vi "Drivetrain Loop.vi"   [LabVIEW 2014]
uses:
  Common Code/Drivetrain Status.ctl
  Drivetrain Mode.ctl
  Common Code/Dist Drive Status.ctl
  Common Code/Yaw Rate Compensation Indicators.ctl
  Common Code/Change Detect Int.vi
  Common Code/Change Detect Boolean.vi
  Robot Global Data.vi
types:
  T1 = typedef "Drivetrain Mode.ctl" = enum16{"Manual", "Gyro Steer", "Vision Steer", "Drive Distance", "Yaw Rate Compensate"}
  T2 = typedef "Drivetrain Status.ctl" = cluster{"Y (Throttle)":sgl, "X (Steer)":sgl, "Translation X":sgl, "Center Wheel Down":bool, "Mode":T1, "Distance Drive finished?":bool, "Y Target":sgl, "X Target":sgl, "Heading Target":sgl, "Dist Drive Status":T3, "Step Eject Lockout":bool, "Gyro In Range?":bool, "Yaw Comp Indicators":T4}
  T3 = typedef "Dist Drive Status.ctl" = cluster{"Y In Range":bool, "X In Range":bool, "Gyro In Range":bool, "Y Dist":dbl, "X Dist":dbl, "Gyro":dbl}
  T4 = typedef "Yaw Rate Compensation Indicators.ctl" = cluster{"Rate Command":sgl, "Rate Actual":sgl, "Steer adjustment":sgl}
  T5 = typedef "Drivetrain Control.ctl" = cluster{"Mode":T1, "Steer":dbl, "Y":dbl, "Heading Target":dbl, "Strafe X":dbl, "Y Target":dbl, "Strafe Target":dbl, "X Max Speed":dbl, "X Min Speed":dbl, "Y Max Speed":dbl, "Y Min Speed":dbl, "Force strafe":bool, "Pivot Speed":dbl}
  T6 = typedef "WPI_DriverStationRobotMode2.ctl" = enum16{"Autonomous Disabled", "Autonomous Enabled", "Teleop Disabled", "Teleop Enabled", "Disconnected", "Finish", "Test Disabled", "Test Enabled", "Emergency Stopped"}
  T7 = typedef "IMU Data.ctl" = cluster{"Pitch":sgl, "Roll":sgl, "Yaw":sgl, "Data Valid?":bool, "Temp":sgl, "MOVING":bool, "NAVX_CAL_STATUS":T8, "NAVX_OP_STATUS":T9, "YAW_STABLE":bool, "Accel X":sgl, "Accel Y":sgl, "Accel Z":sgl, "Accel Magnitude":sgl, "Pitch Rate":sgl, "Roll Rate":sgl, "Yaw Rate":sgl, "NavX Opened?":bool}
  T8 = typedef "navX-MXP IMU.lvlib/navX NAVX_CAL_STATUS.ctl" = u8
  T9 = typedef "navX-MXP IMU.lvlib/navX NAVX_OP_STATUS.ctl" = u8
  T10 = typedef "WPI_MotorControlDeviceRef.ctl" = cluster{"DeviceStatus":errorcluster, "Type":T11, "PWM":cluster{"Controller":T12, "PWM Channel":T13, "DeadBand":T14}, "CAN":cluster{"Device Number":u8, "Control Mode":T15, "Semaphore":T16, "Max Vout":dbl, "TalonSRX Control Mode":T17}, "Invert":bool, "TransformRef":T18, "InvTransformRef":T18}
  T11 = typedef "WPI_MotorControlType.ctl" = enum16{"PWM", "CAN", "CANTalonSRX"}
  T12 = typedef "FPGA_TypedefDigitalModule.ctl" = enum16{"Controller 1"}
  T13 = typedef "FPGA_DIOPWMChannel.ctl" = enum8{"PWM 0", "PWM 1", "PWM 2", "PWM 3", "PWM 4", "PWM 5", "PWM 6", "PWM 7", "PWM 8", "PWM 9", "PWM MXP 0", "PWM MXP 1", "PWM MXP 2", "PWM MXP 3", "PWM MXP 4", "PWM MXP 5", "PWM MXP 6", "PWM MXP 7", "PWM MXP 8", "PWM MXP 9", "Invalid"}
  T14 = typedef "WPI_PWMDeadband.ctl" = cluster{"Name":string, "maxPositivePwm":i32, "minPositivePwm":i32, "centerPwm":i32, "maxNegativePwm":i32, "minNegativePwm":i32, "angularRange":u16}
  T15 = typedef "WPI_CANJaguar_ControlMode.ctl" = enum8{"Percent VBus", "Current", "Speed", "Position", "Voltage"}
  T16 = typedef "Semaphore RefNum" = refnum<k1>
  T17 = typedef "WPI_CANTalonSRX_APIControlMode.ctl" = enum8{"Percent VBus", "Speed", "Position", "Slave", "Unchanged / Invalid"}
  T18 = typedef "WPI_PWMTransform_ConPane.ctl" = refnum<vi>
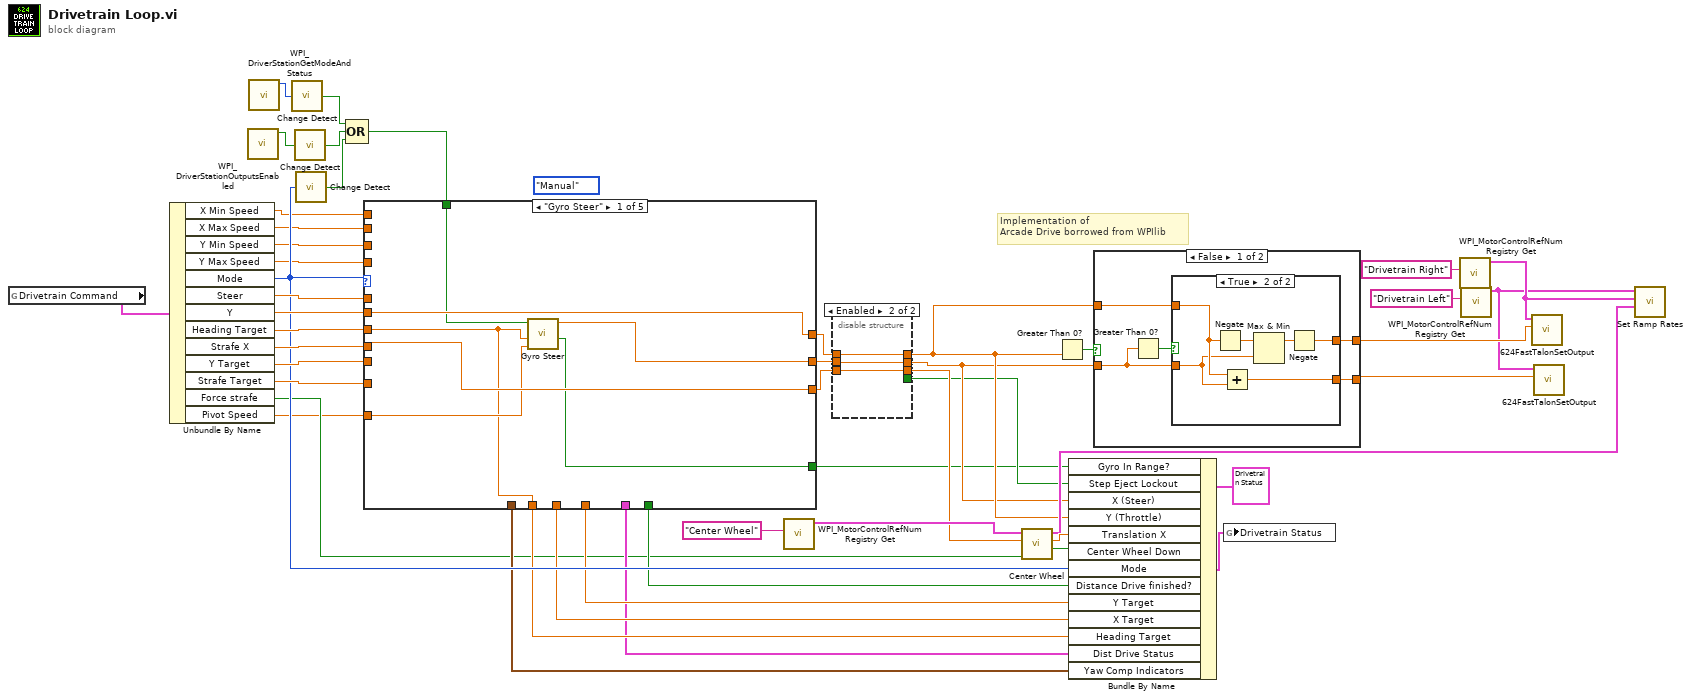
[diagram p0: block diagram]
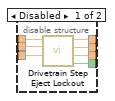
[diagram p2: hidden frame]
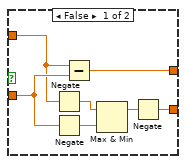
[diagram p3: hidden frame]
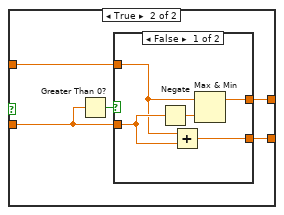
[diagram p4: hidden frame]
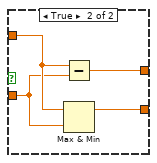
[diagram p5: hidden frame]
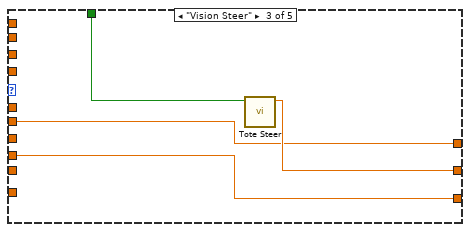
[diagram p7: hidden frame]
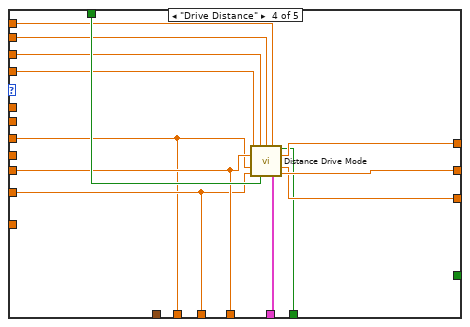
[diagram p8: hidden frame]
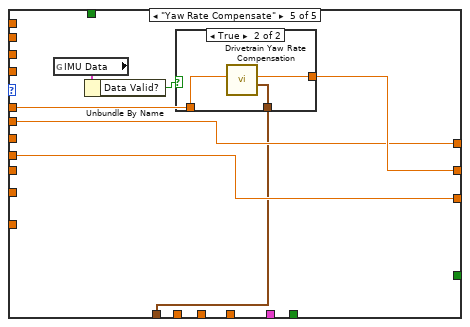
[diagram p9: hidden frame]
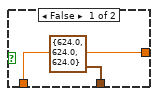
[diagram p10: hidden frame]
diagram:
  (unwired) Drivetrain_Mode."Manual" ("Mode")
  # "Implementation of \nArcade Drive borrowed from WPIlib"
  n1 = global read "Robot Global Data.vi" "Drivetrain Command"() -> (w46:T5)
  n2 = Unbundle By Name(w46) -> ("X Min Speed"=w12:dbl, "X Max Speed"=w13:dbl, "Y Min Speed"=w14:dbl, "Y Max Speed"=w15:dbl, "Mode"=w37:T1, "Steer"=w45:dbl, "Y"=w48:dbl, "Heading Target"=w47:dbl, "Strafe X"=w44:dbl, "Y Target"=w43:dbl, "Strafe Target"=w42:dbl, "Force strafe"=w2:bool, "Pivot Speed"=w1:dbl)
  n3 = call <vilib>:"WPI_DriverStationOutputsEnabled.vi"() -> ("OutputsEnabled?"=w35:bool)  [unwired: 10 in, 1 out]
  n4 = call <vilib>:"WPI_DriverStationGetModeAndStatus.vi"() -> ("Robot Mode"=w36:T6)  [unwired: 10 in, 1 out]
  n5 = call-poly "Change Detect.vi"("In"=w36) -> ("Changed?"=w32:bool)
  n6 = call-poly "Change Detect.vi"("In"=w35) -> ("Changed?"=w33:bool)
  n7 = call-poly "Change Detect.vi"("In"=w37) -> ("Changed?"=w34:bool)
  n8 = Compound Arithmetic op=OR(w32, w33, w34) -> (w31:bool)
  n9 = case shown="\"Gyro Steer\"" w37 {
    tunnel: [w54 w58 w62 w74 w81] -> w9
    tunnel: w45 -> [_ w58 _ _ w82]
    tunnel: [w55 w57 w61 w75 w80] -> w11
    tunnel: w48 -> [w55 w57 w61 _ w80]
    tunnel: w47 -> [w49 _ _ w68 _]
    tunnel: w44 -> [w53 w56 w60 _ w79]
    tunnel: [w53 w56 w60 w73 w79] -> w7
    tunnel: w43 -> [_ _ _ w70 _]
    tunnel: w42 -> [_ _ _ w69 _]
    tunnel: w31 -> [w52 _ w59 w72 _]
    tunnel: [_ _ _ w71 _] -> w30
    tunnel: [_ _ _ w70 _] -> w29
    tunnel: [_ _ _ w69 _] -> w28
    tunnel: [w49 _ _ w68 _] -> w27
    tunnel: [_ _ _ w67 _] -> w26
    tunnel: w15 -> [_ _ _ w66 _]
    tunnel: w14 -> [_ _ _ w65 _]
    tunnel: w13 -> [_ _ _ w64 _]
    tunnel: w12 -> [_ _ _ w63 _]
    tunnel: [w51 _ _ _ _] -> w4
    tunnel: [_ _ _ _ w78] -> w3
    tunnel: w1 -> [w50 _ _ _ _]
    frame "Gyro Steer" {
      n10 = call "Gyro Steer.vi"("Turn Speed"=w50, "Target Angle"=w49, "Changed?"=w52) -> ("In Range?"=w51:bool, "X out"=w54:dbl)  [unwired: 7 in]
    }
    frame "Manual", Default {
    }
    frame "Vision Steer" {
      n11 = call "Tote Steer.vi"("Changed?"=w59) -> ("f"=w62:dbl)  [unwired: 10 in]
    }
    frame "Drive Distance" {
      n12 = call "Distance Drive Mode.vi"("Y Output High"=w66, "Y Output Low"=w65, "X Output High"=w64, "X Output Low"=w63, "Y target"=w70, "Heading target"=w68, "Strafe target"=w69, "Reinitialize"=w72) -> ("isFinished"=w71:bool, "Y out"=w75:dbl, "Strafe out"=w73:dbl, "Dist Drive Status"=w67:T3, "X out"=w74:dbl)  [unwired: 3 in]
    }
    frame "Yaw Rate Compensate" {
      n13 = global read "Robot Global Data.vi" "IMU Data"() -> (w77:T7)
      n14 = Unbundle By Name(w77) -> ("Data Valid?"=w76:bool)
      n15 = case shown="True" w76 {
        tunnel: w82 -> [w84 w87]
        tunnel: [w84 w86] -> w81
        tunnel: [T4 {"Rate Command"=624.0, "Rate Actual"=624.0, "Steer adjustment"=624.0} ("Yaw Comp Indicators") w85] -> w78
        frame False {
        }
        frame True {
          n16 = call "Drivetrain Yaw Rate Compensation.vi"("Steer in"=w87) -> ("Yaw Comp Indicators"=w85:T4, "Steer Out"=w86:dbl)  [unwired: 9 in]
        }
      }
    }
  }
  n17 = call <vilib>:"WPI_MotorControlRefNum Registry Get.vi"("refnum name"="Center Wheel") -> ("MotorControlDevRef"=w19:T10)  [unwired: 9 in, 1 out]
  n18 = disable-structure shown="Enabled" {
    disable-tunnel: w11 -> [w94 w97]
    disable-tunnel: [w93 w97] -> w10
    disable-tunnel: w9 -> [w92 w96]
    disable-tunnel: [w91 w96] -> w8
    disable-tunnel: w7 -> [w90 w95]
    disable-tunnel: [w89 w95] -> w6
    disable-tunnel: [w88 _] -> w5
    frame Disabled {
      n19 = call "Drivetrain Step Eject Lockout.vi"("Strafe In"=w90, "Steer In"=w92, "Throttle In"=w94) -> ("Eject Lockout?"=w88:bool, "Strafe Out"=w89:dbl, "Steer Out"=w91:dbl, "Throttle Out"=w93:dbl)  [unwired: 5 in]
    }
    frame Enabled {
    }
  }
  n20 = call "Center Wheel.vi"("Force strafe"=w2, "Center Wheel Value"=w6, "MotorControlDevRef"=w19) -> ("Wheel Down"=w38:bool, "X Out"=w39:dbl, "MotorControlDevRef 2"=w18:T10)  [unwired: 6 in]
  n21 = Greater Than 0?(x=w10) -> (x > 0?=w25:bool)
  n22 = Bundle By Name(cluster=T2 {"Y (Throttle)"=0.0, "X (Steer)"=0.0, "Translation X"=0.0, "Center Wheel Down"=FALSE, "Mode"=enum."Manual", "Distance Drive finished?"=FALSE, "Y Target"=0.0, "X Target"=0.0, "Heading Target"=0.0, "Dist Drive Status"={"Y In Range"=FALSE, "X In Range"=FALSE, "Gyro In Range"=FALSE, "Y Dist"=0.0, "X Dist"=0.0, "Gyro"=0.0}, "Step Eject Lockout"=FALSE, "Gyro In Range?"=FALSE, "Yaw Comp Indicators"={"Rate Command"=0.0, "Rate Actual"=0.0, "Steer adjustment"=0.0}} ("Drivetrain Status"), "Gyro In Range?"=w4, "Step Eject Lockout"=w5, "X (Steer)"=w8, "Y (Throttle)"=w10, "Translation X"=w39, "Center Wheel Down"=w38, "Mode"=w37, "Distance Drive finished?"=w30, "Y Target"=w29, "X Target"=w28, "Heading Target"=w27, "Dist Drive Status"=w26, "Yaw Comp Indicators"=w3) -> (w41:T2)
  n23 = case shown="False" w25 {
    tunnel: w8 -> [w101 w119]
    tunnel: w10 -> [w100 w118]
    tunnel: [w99 w117] -> w22
    tunnel: [w98 w116] -> w21
    frame False {
      n24 = Greater Than 0?(x=w101) -> (x > 0?=w102:bool)
      n25 = case shown="True" w102 {
        tunnel: w101 -> [w109 w111]
        tunnel: w100 -> [w107 w112]
        tunnel: [w103 w113] -> w99
        tunnel: [w104 w110] -> w98
        frame False {
          n26 = Negate(x=w107) -> (-x=w108:dbl)
          n27 = Negate(x=w109) -> (-x=w106:dbl)
          n28 = Subtract(x=w107, y=w109) -> (x-y=w103:dbl)
          n29 = Max & Min(x=w108, y=w106) -> (max(x,y)=w105:dbl)  [unwired: 1 out]
          n30 = Negate(x=w105) -> (-x=w104:dbl)
        }
        frame True {
          n31 = Negate(x=w112) -> (-x=w115:dbl)
          n32 = Add(x=w112, y=w111) -> (x+y=w110:dbl)
          n33 = Max & Min(x=w115, y=w111) -> (max(x,y)=w114:dbl)  [unwired: 1 out]
          n34 = Negate(x=w114) -> (-x=w113:dbl)
        }
      }
    }
    frame True {
      n35 = Greater Than 0?(x=w119) -> (x > 0?=w120:bool)
      n36 = case shown="False" w120 {
        tunnel: w119 -> [w125 w127]
        tunnel: w118 -> [w122 w128]
        tunnel: [w123 w126] -> w117
        tunnel: [w121 w129] -> w116
        frame False {
          n37 = Negate(x=w125) -> (-x=w124:dbl)
          n38 = Add(x=w122, y=w125) -> (x+y=w121:dbl)
          n39 = Max & Min(x=w122, y=w124) -> (max(x,y)=w123:dbl)  [unwired: 1 out]
        }
        frame True {
          n40 = Subtract(x=w128, y=w127) -> (x-y=w126:dbl)
          n41 = Max & Min(x=w128, y=w127) -> (max(x,y)=w129:dbl)  [unwired: 1 out]
        }
      }
    }
  }
  n42 = global write "Robot Global Data.vi" "Drivetrain Status"(w41) -> ()
  n43 = call <vilib>:"WPI_MotorControlRefNum Registry Get.vi"("refnum name"="Drivetrain Right") -> ("MotorControlDevRef"=w17:T10)  [unwired: 9 in, 1 out]
  n44 = call <vilib>:"WPI_MotorControlRefNum Registry Get.vi"("refnum name"="Drivetrain Left") -> ("MotorControlDevRef"=w16:T10)  [unwired: 9 in, 1 out]
  n45 = call "624FastTalonSetOutput.vi"("Output"=w22, "MotorControlDevRef"=w17) -> ()  [unwired: 8 in, 2 out]
  n46 = call "624FastTalonSetOutput.vi"("Output"=w21, "MotorControlDevRef"=w16) -> ()  [unwired: 8 in, 2 out]
  n47 = call "Set Ramp Rates.vi"("DT Center"=w18, "DT Right"=w17, "DT Left"=w16) -> ()  [unwired: 9 in]
